vi "CreateHTML.vi"(0 "reference in":refnum<class "WebFrontPanel.lvclass">, 5 "error in (no error)":errorcluster, 7 "Refresh rate (250ms)":i32=250) -> (12 "Name":string, 14 "reference out":refnum<class "WebFrontPanel.lvclass">, 15 "HTML":string, 16 "js":string, 19 "error out":errorcluster)   [LabVIEW 2014, in "FrontPanelPublisher.lvlib" / "WebFrontPanel.lvclass"]
uses:
  WebFrontPanel.lvclass
  Controls/HTMLTemplateFill.ctl
  Controls/JSTemplateFill.ctl
  <userlib>/_OpenG.lib/array/array.llb/Remove Duplicates from 1D Array (String)__ogtk.vi
  Object_class/Object.lvclass
  FrontPanelManager_class/FrontPanelManager.lvclass
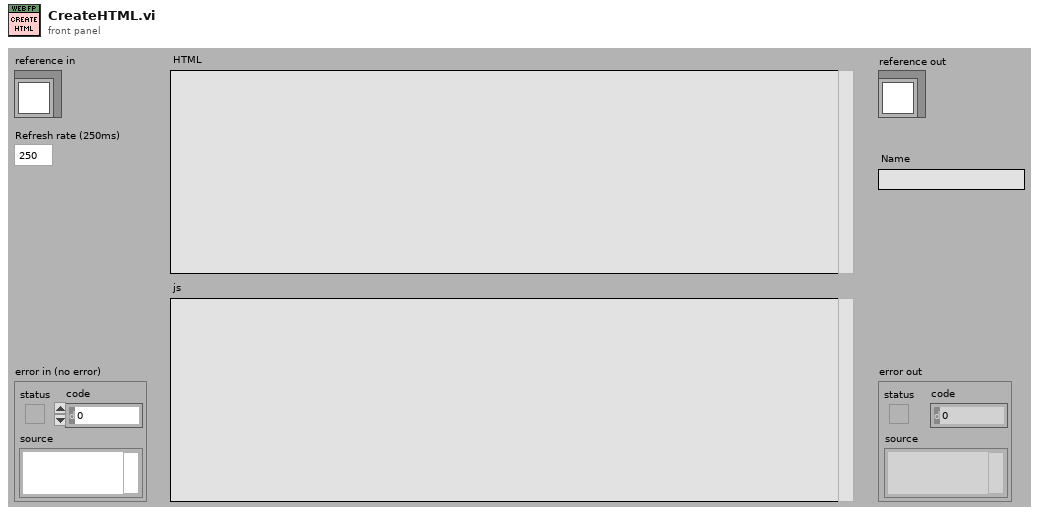
[diagram p1: front panel]
types:
  T1 = typedef "FrontPanelPublisher.lvlib/WebFrontPanel.lvclass/JSTemplateFill.ctl" = cluster{"Page Name":string, "js varibles":string, "Code for controls":string, "Code for indicators":string, "Refresh rate (ms)":i32}
  T2 = typedef "FrontPanelPublisher.lvlib/WebFrontPanel.lvclass/HTMLTemplateFill.ctl" = cluster{"Page Name":string, "Script dependencies":string, "Body width (px)":i32, "Body height (px)":i32, "Background Colour":u32, "HTML elements":string}
  T3 = typedef "FrontPanelPublisher.lvlib/WebFrontPanel.lvclass/ObjectAttributes.ctl" = cluster{"VI Name":string, "VI Reference":refnum<vi>, "Controls":refnum<class "Object.lvclass">[], "Indicators":refnum<class "Object.lvclass">[], "Decorations":refnum<class "Object.lvclass">[]}
  T4 = typedef "LVRectTypeDef.ctl" = cluster{"Left":i16, "Top":i16, "Right":i16, "Bottom":i16}
  T5 = typedef "FrontPanelPublisher.lvlib/FrontPanelManager.lvclass/WebsocketInfo.ctl" = cluster{"Hostname":string, "Port":u16}
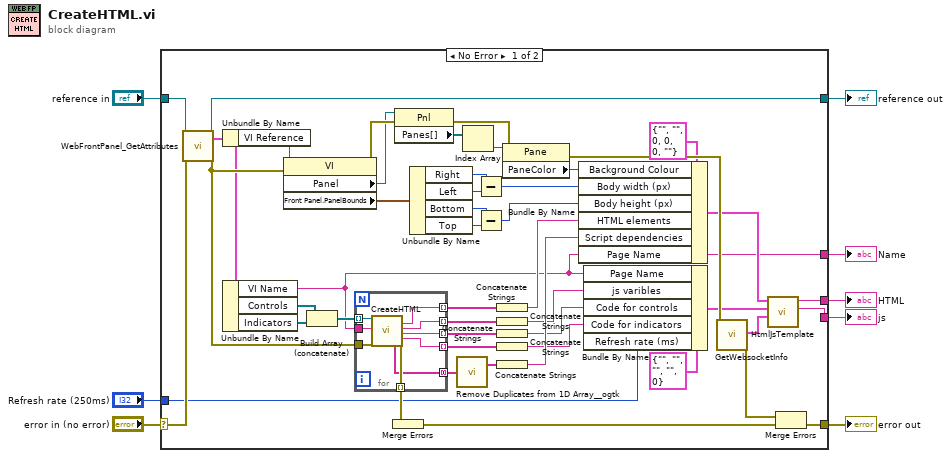
[diagram p0: block diagram]
diagram:
  n1 = case shown="No Error" "error in (no error)" {
    selector: "error in (no error)" -> [w55 w66]
    tunnel: [w50 w66] -> w7
    tunnel: [w46 w65] -> w5
    tunnel: "reference in" -> [w47 w65]
    tunnel: [w27 _] -> w3
    tunnel: "Refresh rate (250ms)" -> [w10 _]
    tunnel: [w11 _] -> w2
    tunnel: [w13 _] -> w1
    frame No Error {
      n2 = call "WebFrontPanel_GetAttributes.vi"("reference in"=w47, "error in (no error)"=w55) -> ("reference out"=w46:refnum<class "WebFrontPanel.lvclass">, "Data"=w31:T3, "error out"=w53:errorcluster)  [unwired: 14 in, 1 out]
      n3 = Unbundle By Name(w31) -> ("VI Reference"=w35:refnum<vi>)
      n4 = Unbundle By Name(w31) -> ("VI Name"=w13:string, "Controls"=w30:refnum<class "Object.lvclass">[], "Indicators"=w29:refnum<class "Object.lvclass">[])
      n5 = property class="VI"(reference=w35, error in=w53) -> (error out=w52:errorcluster, "Panel"=w20:refnum<vi>, "Front Panel.PanelBounds"=w40:T4)  [unwired: 1 out]
      n6 = Build Array (concatenate)(w30, w29) -> (w32:refnum<class "Object.lvclass">[])
      n7 = for {
        tunnel: w32 -> [w62] mode=indexing
        tunnel: [w61] -> w45 mode=indexing
        tunnel: [w60] -> w44 mode=indexing
        tunnel: [w59] -> w43 mode=indexing
        tunnel: [w58] -> w42 mode=concatenating
        tunnel: w53 -> [w64]
        tunnel: [w63] -> w34 mode=indexing
        tunnel: [w57] -> w33 mode=indexing
        tunnel: w13 -> [w56]
        n8 = call-dynamic "CreateHTML.vi"("reference in"=w62, "VI Name"=w56, "error in (no error)"=w64) -> ("script dependencies"=w58:string[], "HTML"=w61:string, "js variables"=w60:string, "js code for controls"=w59:string, "js code for indicators"=w57:string, "error out"=w63:errorcluster)  [unwired: 10 in, 1 out]
      }
      n9 = Merge Errors(w34) -> (w54:errorcluster)
      n10 = property class="Pnl"(reference=w20, error in=w52) -> (error out=w51:errorcluster, "Panes[]"=w22:refnum<vi>[])  [unwired: 1 out]
      n11 = Unbundle By Name(w40) -> ("Right"=w39:i16, "Left"=w38:i16, "Bottom"=w37:i16, "Top"=w36:i16)
      n12 = call-poly <userlib>:"Remove Duplicates from 1D Array__ogtk.vi"("Input Array"=w42) -> ("Output Array"=w41:string[])  [unwired: 1 out]
      n13 = Index Array(array=w22) -> (element=w21:refnum<vi>)  [unwired: 1 in]
      n14 = Subtract(x=w39, y=w38) -> (x-y=w26:i16)
      n15 = Subtract(x=w37, y=w36) -> (x-y=w25:i16)
      n16 = Concatenate Strings(w45) -> (w24:string)
      n17 = Concatenate Strings(w44) -> (w16:string)
      n18 = Concatenate Strings(w43) -> (w15:string)
      n19 = Concatenate Strings(w33) -> (w14:string)
      n20 = Concatenate Strings(w41) -> (w23:string)
      n21 = property class="Pane"(reference=w21, error in=w51) -> (error out=w49:errorcluster, "PaneColor"=w19:u32)  [unwired: 1 out]
      n22 = Bundle By Name(cluster=T2 {"Page Name"="", "Script dependencies"="", "Body width (px)"=0, "Body height (px)"=0, "Background Colour"=0, "HTML elements"=""} ("HTML"), "Background Colour"=w19, "Body width (px)"=w26, "Body height (px)"=w25, "HTML elements"=w24, "Script dependencies"=w23, "Page Name"=w13) -> (w18:T2)
      n23 = Bundle By Name(cluster=T1 {"Page Name"="", "js varibles"="", "Code for controls"="", "Code for indicators"="", "Refresh rate (ms)"=0} ("js"), "Page Name"=w13, "js varibles"=w16, "Code for controls"=w15, "Code for indicators"=w14, "Refresh rate (ms)"=w10) -> (w12:T1)
      n24 = call "GetWebsocketInfo.vi"("error in (no error)"=w49) -> ("Websocket Info"=w9:T5, "error out"=w48:errorcluster)  [unwired: 17 in]
      n25 = call "HtmlJsTemplate.vi"("Websocket Info"=w9, "js"=w12, "HTML"=w18) -> ("js out"=w11:string, "HTML out"=w27:string)  [unwired: 7 in]
      n26 = Merge Errors(w48, w54) -> (w50:errorcluster)
    }
    frame Error {
    }
  }
  "error out" <- w7
  "reference out" <- w5
  "HTML" <- w3
  "js" <- w2
  "Name" <- w1
